vi "Add Child.vi"(4 "Position":i32[](array[numeric]), 6 "Tree Item In":T1, 8 "error in (no error)":errorcluster, 9 "Data In":refnum<class "Tree Data.lvclass">, 10 "Tree In":refnum<class "Tree.lvclass">, 11 "Tree Data in":refnum<class "Tree Data.lvclass">) -> (0 "error out":errorcluster, 2 "Tree Out":refnum<class "Tree.lvclass">, 3 "Tree Data out":refnum<class "Tree Data.lvclass">)   [LabVIEW 2022 SP3, in "Tree Data.lvclass"]
uses:
  Tree Data.lvclass
  Tree/Tree.lvclass
  Tree/Type Def/Tree Item.ctl
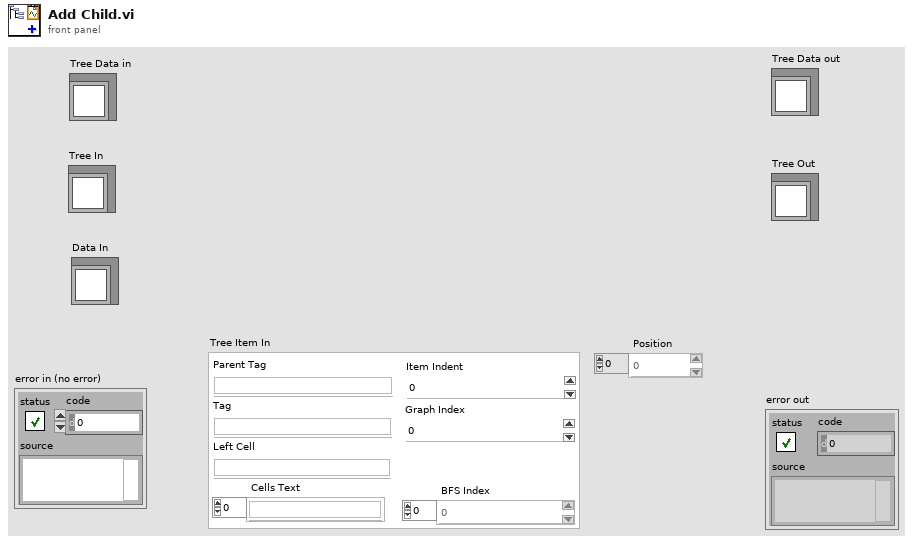
[diagram p1: front panel]
types:
  T1 = typedef "Tree Item.ctl" = cluster{"Parent Tag":string, "Tag":string, "Left Cell":string, "Cells Text":string[], "BFS Index":i32[], "Graph Index":i32, "Item Indent":i32}
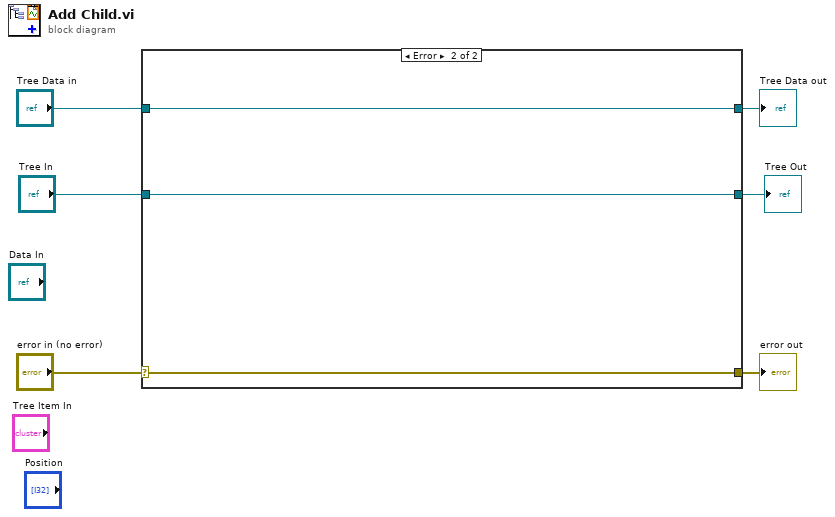
[diagram p0: block diagram]
diagram:
  n1 = case shown="Error" "error in (no error)" {
    selector: "error in (no error)" -> [w8 w12]
    tunnel: [w8 w12] -> w5
    tunnel: [w9 w11] -> w3
    tunnel: "Tree Data in" -> [w9 w11]
    tunnel: [w7 w10] -> w2
    tunnel: "Tree In" -> [w7 w10]
    frame No Error {
      # "Wire the error cluster across even in the \"No Error\"\ncase so that warnings get propagated."
    }
    frame Error {
    }
  }
  "error out" <- w5
  "Tree Data out" <- w3
  "Tree Out" <- w2
